vi "Child Text.vi"(8 "Error In":errorcluster, 10 "Label Text":string, 11 "Bookmark Tag":string) -> (0 "Error Out":errorcluster, 3 "Child Text":string[](array[string]))   [LabVIEW 2017, in "Bookmark Manager.lvlib"]
uses:
  Bookmark Manager.lvlib
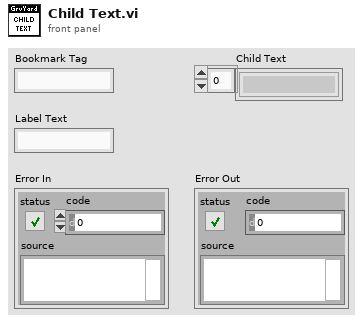
[diagram p1: front panel]
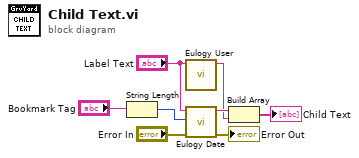
[diagram p0: block diagram]
diagram:
  n1 = String Length(string="Bookmark Tag") -> (length=w8:i32)
  n2 = call "Eulogy User.vi"("Label Text"="Label Text") -> ("User"=w3:string)  [unwired: 10 in]
  n3 = call "Eulogy Date.vi"("Error In"="Error In", "Tag Length"=w8, "Label Text"="Label Text") -> ("Error Out"=→"Error Out":errorcluster, "Date"=w6:string)  [unwired: 7 in]
  n4 = Build Array(w6, w3) -> (→"Child Text":string[])
